vi "Config file.vi"(6 "path":path, 7 "access (0:read/write)":enum16{"read/write", "read-only", "write-only"}(ring), 8 "error in (no error)":errorcluster, 9 "data values":variant[](array[variant]), 11 "email settings":T1) -> (0 "error out":errorcluster, 1 "data out":variant[](array[variant]))   [LabVIEW 2018]
uses:
  <vilib>/Utility/xml.llb/Write to XML File(string).vi
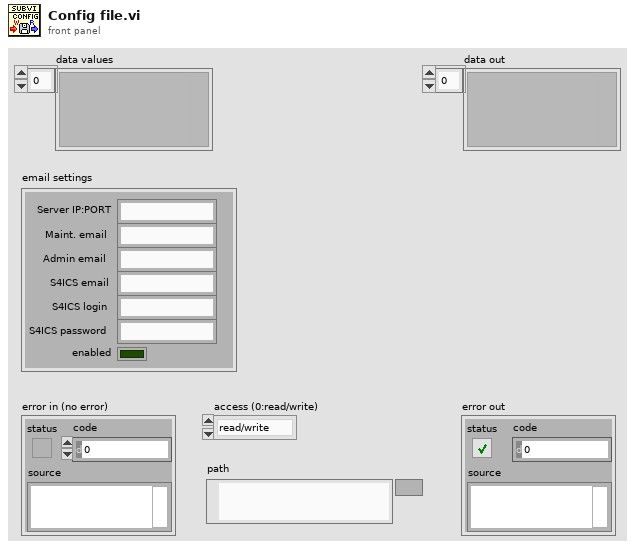
[diagram p1: front panel]
types:
  T1 = cluster{"email service":string, "maint. email":string, "admin email":string, "S4ICS email":string, "S4ICS login":string, "S4ICS password":string, "email enabled":bool}
  T2 = enum16{"open", "replace", "create", "open or create", "replace or create", "replace or create with confirmation"}
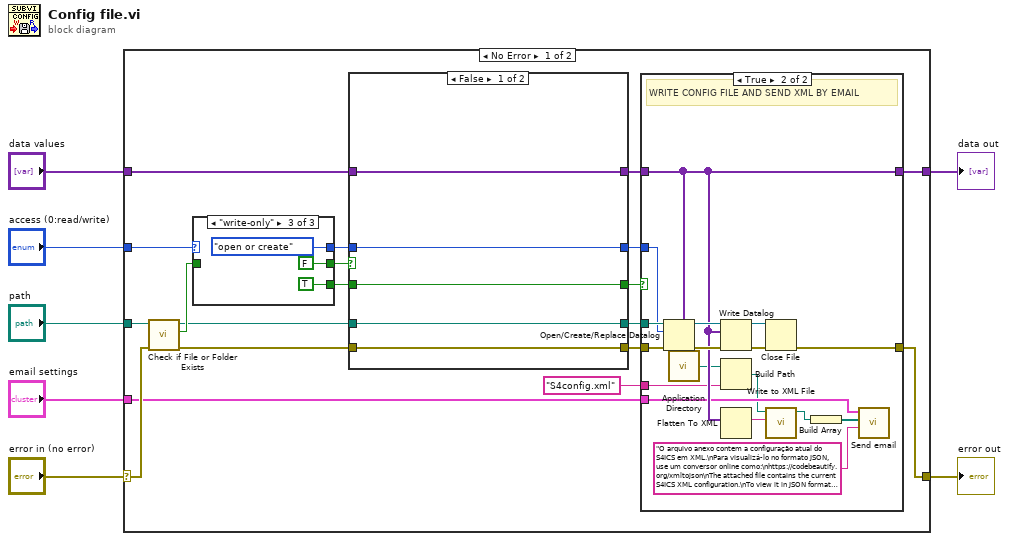
[diagram p0: block diagram]
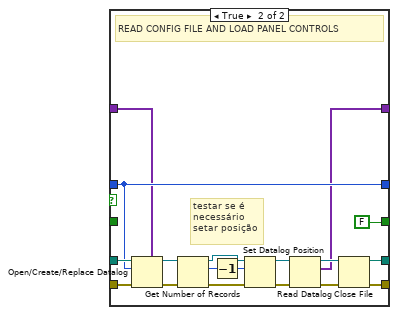
[diagram p3: hidden frame]
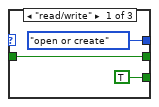
[diagram p4: hidden frame]
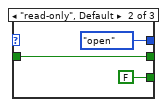
[diagram p5: hidden frame]
diagram:
  n1 = case shown="No Error" "error in (no error)" {
    selector: "error in (no error)" -> [w25 w79]
    tunnel: "path" -> [w24 _]
    tunnel: "access (0:read/write)" -> [w23 _]
    tunnel: "data values" -> [w14 w78]
    tunnel: [w11 w78] -> w3
    tunnel: "email settings" -> [w9 _]
    tunnel: [w10 w79] -> w1
    frame No Error {
      n2 = call <vilib>:"Check if File or Folder Exists.vi"("error in (no error)"=w25, "path"=w24) -> ("error out"=w18:errorcluster, "file or folder exists?"=w26:bool, "dup path"=w19:path)  [unwired: 7 in]
      n3 = case shown="\"write-only\"" w23 {
        tunnel: [w71 w74 FALSE] -> w22
        tunnel: w26 -> [w71 w74 _]
        tunnel: [TRUE FALSE TRUE] -> w20
        tunnel: [T2."open or create" ("operation (0:open)") T2."open" ("operation (0:open)") T2."open or create" ("operation (0:open)")] -> w17
        frame "read/write" {
        }
        frame "read-only", Default {
        }
        frame "write-only" {
        }
      }
      n4 = case shown="False" w22 {
        tunnel: [w50 FALSE] -> w21
        tunnel: w20 -> [w50 _]
        tunnel: w19 -> [w46 w67]
        tunnel: w18 -> [w47 w66]
        tunnel: w17 -> [w49 w65]
        tunnel: [w49 w65] -> w16
        tunnel: [w47 w60] -> w15
        tunnel: w14 -> [w48 w58]
        tunnel: [w48 w52] -> w12
        tunnel: [w46 w51] -> w13
        frame False {
        }
        frame True {
          # "testar se é\nnecessário\nsetar posição"
          # "READ CONFIG FILE AND LOAD PANEL CONTROLS"
          n5 = Open/Create/Replace Datalog(5:w58, 8:w66, 10:w65, 11:w67) -> (0:w61:errorcluster, 3:w59:refnum<k1>)  [unwired: 2 in, 1 out]
          n6 = Get Number of Records(4:w61, 7:w59) -> (0:w64:errorcluster, 2:w56:i64, 3:w57:refnum<k1>)
          n7 = Decrement(x=w56) -> (x-1=w55:i64)
          n8 = Set Datalog Position(4:w64, 6:w55, 7:w57) -> (0:w63:errorcluster, 3:w54:refnum<k1>)  [unwired: 1 in]
          n9 = Read Datalog(4:w63, 7:w54) -> (0:w62:errorcluster, 2:w52:variant[], 3:w53:refnum<k1>)  [unwired: 1 in]
          n10 = Close File(refnum=w53, error in=w62) -> (path=w51:path, error out=w60:errorcluster)
        }
      }
      n11 = case shown="True" w21 {
        tunnel: w16 -> [_ w29]
        tunnel: w15 -> [w27 w45]
        tunnel: w13 -> [_ w41]
        tunnel: [w27 w42] -> w10
        tunnel: w12 -> [w28 w38]
        tunnel: [w28 w38] -> w11
        tunnel: w9 -> [_ w33]
        tunnel: "S4config.xml" ("string") -> [_ w31]
        frame False {
        }
        frame True {
          # "WRITE CONFIG FILE AND SEND XML BY EMAIL"
          n12 = Open/Create/Replace Datalog(5:w38, 8:w45, 10:w29, 11:w41) -> (0:w44:errorcluster, 3:w40:refnum<k1>)  [unwired: 2 in, 1 out]
          n13 = call <vilib>:"Application Directory.vi"() -> ("Application Directory"=w32:path)
          n14 = Write Datalog(4:w44, 6:w38, 7:w40) -> (0:w43:errorcluster, 3:w39:refnum<k1>)
          n15 = Build Path(base path=w32, name or relative path=w31) -> (appended path=w30:path)
          n16 = Flatten To XML(anything=w38) -> (xml string=w37:string)
          n17 = Close File(refnum=w39, error in=w43) -> (error out=w42:errorcluster)  [unwired: 1 out]
          n18 = call-poly <vilib>:"Write to XML File.vi"("XML Input"=w37, "XML File Path"=w30) -> ("XML File Path(duplicate)"=w35:path)  [unwired: 7 in, 2 out]
          n19 = Build Array(w35) -> (w36:path[])
          n20 = call "Send email.vi"("message"="O arquivo anexo contem a configuração atual do S4ICS em XML.\nPara visualizá-lo no formato JSON, use um conversor online como:\nhttps://codebeautify.org/xmltojson\nThe attached file contains the current S4ICS XML configuration.\nTo view it in JSON format, use an online converter such as above.", "attachments"=w36, "email settings"=w33) -> ()  [unwired: 7 in, 2 out]
        }
      }
    }
    frame Error {
    }
  }
  "data out" <- w3
  "error out" <- w1
